vi "Element Init.vi"(7 "VolatusAPI":refnum<class "VolatusAPI.lvclass">, 8 "error in (no error)":errorcluster, 10 "JSON":string, 11 "2WayValve in":refnum<class "2WayValveV.lvclass">) -> (0 "error out":errorcluster, 3 "2WayValve out":refnum<class "2WayValveV.lvclass">)   [LabVIEW 2023, in "VolatusGUIElements.lvlib" / "2WayValveV.lvclass"]
uses:
  2WayValveV.lvclass
  C:/dev/volatus/mts-volatus-super/libs/lv-volatus/VolatusGUI/GUI Element/GUI Element.lvclass
  Volatus/VolatusAPI/VolatusAPI.lvclass
  JSON.ctl
  Group Channel.ctl
  Unused Element.ctl
  Values.ctl
  Channel State.ctl
  VolatusGUI/GUI Element/GUI Element.lvclass/GUI Element.ctl
  lv-vecto/Vecto/Group DBL/Group DBL.lvclass
  C:/dev/volatus/mts-volatus-super/libs/lv-vecto/Vecto/Group/Group.lvclass
  lv-vecto/Vecto/Channel DBL/Channel DBL.lvclass/Channel DBL.ctl
  2WayValveV.lvclass/2WayValveV.ctl
  5ca493e1-1c63-4061-b4b4-46184d61fbe0.vi
  <vilib>/JDP Science/JSONtext/JSON text to Variant.vi
  lv-vecto/Vecto/Group/Channel Info by Index.vi
  <vilib>/JDP Science/JSONtext/LVClass Serializer/JSONtext LVClass Serializer.lvclass
  lv-vecto/Vecto/Channel DBL/Channel DBL.lvclass
  Volatus/Digital Command/Digital Command.lvclass
  VolatusGUI/Element Inhibit/Element Inhibit.lvclass
  VolatusGUI/GUI Element/GUI Element.lvclass
  VolatusErrorUtilities/MultiErrors/MultiErrors.lvclass
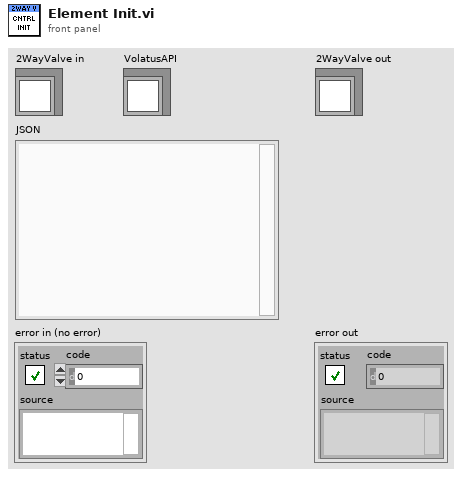
[diagram p1: front panel]
types:
  T1 = typedef "VolatusGUIElements.lvlib/2WayValveV.lvclass/Values.ctl" = cluster{"Command":T2, "CmdFB":T2, "Closed":T2, "Open":T2, "Energized":T2}
  T2 = typedef "VolatusGUIElements.lvlib/2WayValveV.lvclass/Channel State.ctl" = cluster{"Value":bool, "Stale":bool, "Config":bool, "Error":bool, "Prev":bool}
  T3 = typedef "VolatusGUIElements.lvlib/2WayValveV.lvclass/Unused Element.ctl" = cluster{"Command":bool, "Feedback":bool, "Energized":bool}
  T4 = typedef "VolatusGUIElements.lvlib/2WayValveV.lvclass/JSON.ctl" = cluster{"Output":T5, "ClosedFB":T5, "OpenFB":T5, "Energized":cluster{"Channel":string, "Threshold":dbl}, "Staleness":dbl, "Inhibit":string}
  T5 = typedef "VolatusGUIElements.lvlib/2WayValveV.lvclass/Group Channel.ctl" = cluster{"Channel":string}
  T6 = typedef "VectoConfig.lvlib/Channel Info.ctl" = cluster{"Name":string, "Group":string, "Owning Node":string, "Owning Task":string, "Resource":string}
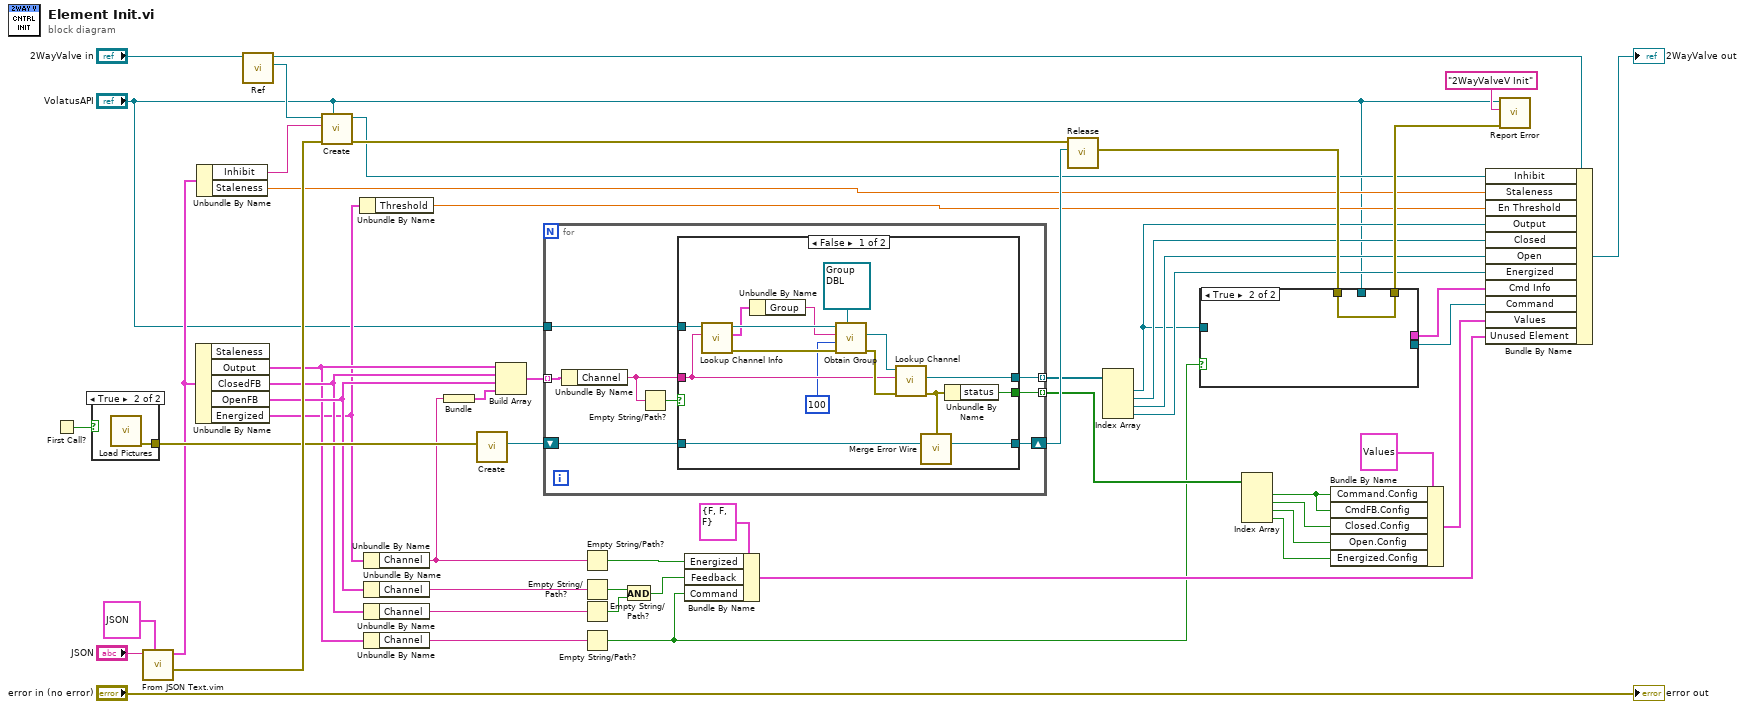
[diagram p0: block diagram]
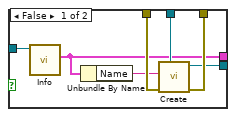
[diagram p2: hidden frame]
diagram:
  n1 = First Call?() -> (First Call?: T/F=w25:bool)
  n2 = case shown="True" w25 {
    tunnel: [_ w54] -> w49
    frame False {
    }
    frame True {
      n3 = call "Load Pictures.vi"() -> ("error out"=w54:errorcluster)  [unwired: 11 in]
    }
  }
  n4 = call "From JSON Text.vim"("Data Type and Default Value"=T4 {"Output"={"Channel"=""}, "ClosedFB"={"Channel"=""}, "OpenFB"={"Channel"=""}, "Energized"={"Channel"="", "Threshold"=0.0}, "Staleness"=0.0, "Inhibit"=""} ("JSON"), "JSON"="JSON") -> ("error out"=w50:errorcluster, "Data out"=w15:T4)  [unwired: 8 in]
  n5 = Unbundle By Name(w15) -> ("Output"=w24:T5, "ClosedFB"=w45:T5, "OpenFB"=w46:T5, "Energized"=w20:cluster{"Channel":string, "Threshold":dbl})  [unwired: 1 out]
  n6 = Unbundle By Name(w15) -> ("Inhibit"=w13:string, "Staleness"=w14:dbl)
  n7 = call "Ref.vi"("GUI Element in"="2WayValve in") -> ("Ref"=w18:refnum<vi>, "GUI Element out"=w16:refnum<class "2WayValveV.lvclass">)  [unwired: 9 in]
  n8 = call "Create.vi"("VolatusAPI"="VolatusAPI", "error in (no error)"=w50, "Inhibit Channel"=w13, "Control Ref"=w18) -> ("error out"=w12:errorcluster, "Element Inhibit out"=w10:refnum<class "Element Inhibit.lvclass">)  [unwired: 6 in]
  n9 = Unbundle By Name(w20) -> ("Threshold"=w19:dbl)
  n10 = Unbundle By Name(w20) -> ("Channel"=w22:string)
  n11 = Unbundle By Name(w46) -> ("Channel"=w44:string)
  n12 = Unbundle By Name(w45) -> ("Channel"=w43:string)
  n13 = Unbundle By Name(w24) -> ("Channel"=w42:string)
  n14 = Bundle("Channel"=w22) -> (w21:cluster{"Channel":string})  [unwired: 1 in]
  n15 = call "Create.vi"("error in (no error)"=w49) -> ("MultiErrors out"=w8:refnum<class "MultiErrors.lvclass">)  [unwired: 10 in]
  n16 = Build Array(w24, w45, w46, w21) -> (w7:T5[])
  n17 = for {
    tunnel: w7 -> [w61] mode=indexing
    tunnel: [w60] -> w6 mode=indexing
    tunnel: [w59] -> w5 mode=indexing
    tunnel: "VolatusAPI" -> [w62]
    shift-right: [w55] -> w51
    shift-left: w8 -> [w56]
    n18 = Unbundle By Name(w61) -> ("Channel"=w58:string)
    n19 = Empty String/Path?(string/path=w58) -> (empty?=w57:bool)
    n20 = case shown="False" w57 {
      tunnel: w62 -> [w76 _]
      tunnel: [w75 _] -> w60
      tunnel: [w74 _] -> w59
      tunnel: w58 -> [w70 _]
      tunnel: w56 -> [w69 w78]
      tunnel: [w64 w78] -> w55
      frame False {
        n21 = call "Lookup Channel Info.vi"("Channel Name"=w70, "VolatusAPI in"=w76) -> ("error out"=w65:errorcluster, "Channel Info"=w72:T6, "VolatusAPI out"=w73:refnum<class "VolatusAPI.lvclass">)  [unwired: 5 in, 2 out]
        n22 = Unbundle By Name(w72) -> ("Group"=w71:string)
        n23 = call "Obtain Group.vi"("Group Type (Abstract)"=refnum<class "Group DBL.lvclass"> refnum ("Vecto.lvlib:Group.lvclass"), "error in (no error)"=w65, "Timeout ms (5000)"=u32 100, "Group Name"=w71, "VolatusAPI in"=w73) -> ("error out"=w77:errorcluster, "Group"=w66:refnum<class "Group DBL.lvclass">)  [unwired: 4 in, 1 out]
        n24 = call "Lookup Channel.vi"("error in (no error)"=w77, "Channel Name"=w70, "Group in"=w66) -> ("error out"=w68:errorcluster, "Channel"=w75:refnum<class "Channel DBL.lvclass">)  [unwired: 6 in, 1 out]
        n25 = call "Merge Error Wire.vi"("error in (no error)"=w68, "MultiErrors in"=w69) -> ("MultiErrors out"=w64:refnum<class "MultiErrors.lvclass">)  [unwired: 13 in]
        n26 = Unbundle By Name(w68) -> ("status"=w74:bool)
      }
      frame True {
      }
    }
  }
  n27 = Empty String/Path?(string/path=w22) -> (empty?=w40:bool)
  n28 = Empty String/Path?(string/path=w44) -> (empty?=w39:bool)
  n29 = Empty String/Path?(string/path=w43) -> (empty?=w38:bool)
  n30 = Empty String/Path?(string/path=w42) -> (empty?=w1:bool)
  n31 = And(x=w39, y=w38) -> (x .and. y?=w37:bool)
  n32 = Bundle By Name(cluster=T3 {"Command"=FALSE, "Feedback"=FALSE, "Energized"=FALSE} ("Unused Element"), "Energized"=w40, "Feedback"=w37, "Command"=w1) -> (w27:T3)
  n33 = call "Release.vi"("MultiErrors in"=w51, "Upstream Error (None)"=w12) -> ("error out"=w52:errorcluster)  [unwired: 9 in]
  n34 = Index Array(array=w6) -> (element #1=w23:refnum<class "Channel DBL.lvclass">, element #2=w31:refnum<class "Channel DBL.lvclass">, element #3=w30:refnum<class "Channel DBL.lvclass">, element #4=w29:refnum<class "Channel DBL.lvclass">)  [unwired: 4 in]
  n35 = case shown="True" w1 {
    tunnel: [w85 w86] -> w53
    tunnel: w52 -> [w84 w86]
    tunnel: w23 -> [w83 _]
    tunnel: [w81 _] -> w4
    tunnel: "VolatusAPI" -> [w80 _]
    tunnel: [w79 _] -> w2
    frame False {
      n36 = call "Info.vi"("Channel in"=w83) -> ("Info"=w79:T6)  [unwired: 8 in, 2 out]
      n37 = Unbundle By Name(w79) -> ("Name"=w82:string)
      n38 = call "Create.vi"("VolatusAPI"=w80, "error in (no error)"=w84, "Channel"=w82) -> ("error out"=w85:errorcluster, "Digital Command out"=w81:refnum<class "Digital Command.lvclass">)  [unwired: 7 in]
    }
    frame True {
    }
  }
  n39 = Index Array(array=w5) -> (element #1=w35:bool, element #2=w34:bool, element #3=w33:bool, element #4=w32:bool)  [unwired: 4 in]
  n40 = Bundle By Name(cluster=T1 {"Command"={"Value"=FALSE, "Stale"=FALSE, "Config"=FALSE, "Error"=FALSE, "Prev"=FALSE}, "CmdFB"={"Value"=FALSE, "Stale"=FALSE, "Config"=FALSE, "Error"=FALSE, "Prev"=FALSE}, "Closed"={"Value"=FALSE, "Stale"=FALSE, "Config"=FALSE, "Error"=FALSE, "Prev"=FALSE}, "Open"={"Value"=FALSE, "Stale"=FALSE, "Config"=FALSE, "Error"=FALSE, "Prev"=FALSE}, "Energized"={"Value"=FALSE, "Stale"=FALSE, "Config"=FALSE, "Error"=FALSE, "Prev"=FALSE}} ("Values"), "Command.Config"=w35, "CmdFB.Config"=w35, "Closed.Config"=w34, "Open.Config"=w33, "Energized.Config"=w32) -> (w28:T1)
  n41 = Bundle By Name(cluster=w16, "Inhibit"=w10, "Staleness"=w14, "En Threshold"=w19, "Output"=w23, "Closed"=w31, "Open"=w30, "Energized"=w29, "Cmd Info"=w2, "Command"=w4, "Values"=w28, "Unused Element"=w27) -> (→"2WayValve out":refnum<class "2WayValveV.lvclass">)
  n42 = call "Report Error.vi"("error in (no error)"=w53, "Context"="2WayValveV Init", "VolatusAPI in"="VolatusAPI") -> ()  [unwired: 7 in, 2 out]
  "error out" <- "error in (no error)"
